vi "AlliGator Compute Interpolated Color Map (Multipoints).vi"(7 "Background Color":u32(colorbox), 8 "Error In":errorcluster, 9 "Decay Range Exponent":dbl=1.0, 10 "Color Array":u32[](array[numeric]), 11 "XY Graph":refnum<vi>) -> (0 "Error Out":errorcluster, 3 "Vertices":cluster{"X":dbl, "Y":dbl}[](array[cluster]))   [LabVIEW 2021, in "AlliGator Phasor Plot Color Map.lvlib"]
doc: "Computes a color map based on user-provided parameters."
uses:
  <vilib>/Utility/error.llb/DialogType.ctl
  <vilib>/picture/picture.llb/imagedata.ctl
  <vilib>/Analysis/geometry.llb/Point in Polygon (Scalar).vi
  AlliGator Phasor Plot Color Map.lvlib
  Image/Image.lvlib
  <vilib>/vision/NI_Vision_Development_Module.lvlib
  <vilib>/Analysis/NI_AAL_Geometry.lvlib
  Time/Time.lvlib
panel:
  out "CPU (s)":dbl
  # "see the AlliGator License on the block diagram (Ctrl+E or Window:Show Block Diagram)"
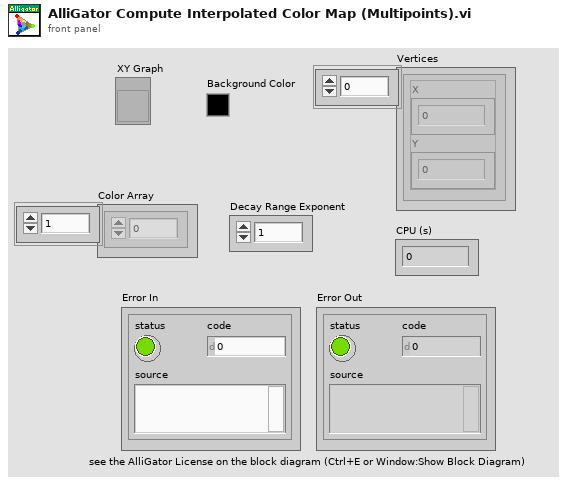
[diagram p1: front panel]
types:
  T1 = typedef "LVCursorListTypeDef.ctl" = cluster{"Name":string, "Color":u32, "Style":u8, "Point Style":u8, "Name Visible":bool, "Allow Drag":bool, "Cursor Mode":u32, "Plot":i32, "Index":i32, "Position":cluster{"X":dbl, "Y":dbl}, "X Scale":u32, "Y Scale":u32, "Watch Plots":i32[], "Watch All Plots":bool, "Plot Area":i32, "Label Offset":cluster{"X":dbl, "Y":dbl}}[]
  T2 = typedef "LVBoundsTypeDef.ctl" = cluster{"Width":u32, "Height":u32}
  T3 = typedef "LVRectTypeDef.ctl" = cluster{"Left":i16, "Top":i16, "Right":i16, "Bottom":i16}
  T4 = cluster{"left":i16, "top":i16, "right":i16, "bottom":i16}
  T5 = typedef "imagedata.ctl" = cluster{"image type":i32, "image depth":i32, "image":u8[], "mask":u8[], "colors":u32[], "Rectangle":cluster{"left":i16, "top":i16, "right":i16, "bottom":i16}}
  T6 = typedef "DialogType.ctl" = u16
  T7 = typedef "LVPoint32TypeDef.ctl" = cluster{"Horizontal":i32, "Vertical":i32}
  T8 = cluster{"Red (or Hue) value":u8, "Green (or Sat) value":u8, "Blue (or Light or Val) value":u8}[]
  T9 = typedef "NI_AAL_Geometry.lvlib/Point in Polygon Position.ctl" = u16
  T10 = cluster{"Red (or Hue) value":u8, "Green (or Sat) value":u8, "Blue (or Light or Val) value":u8}
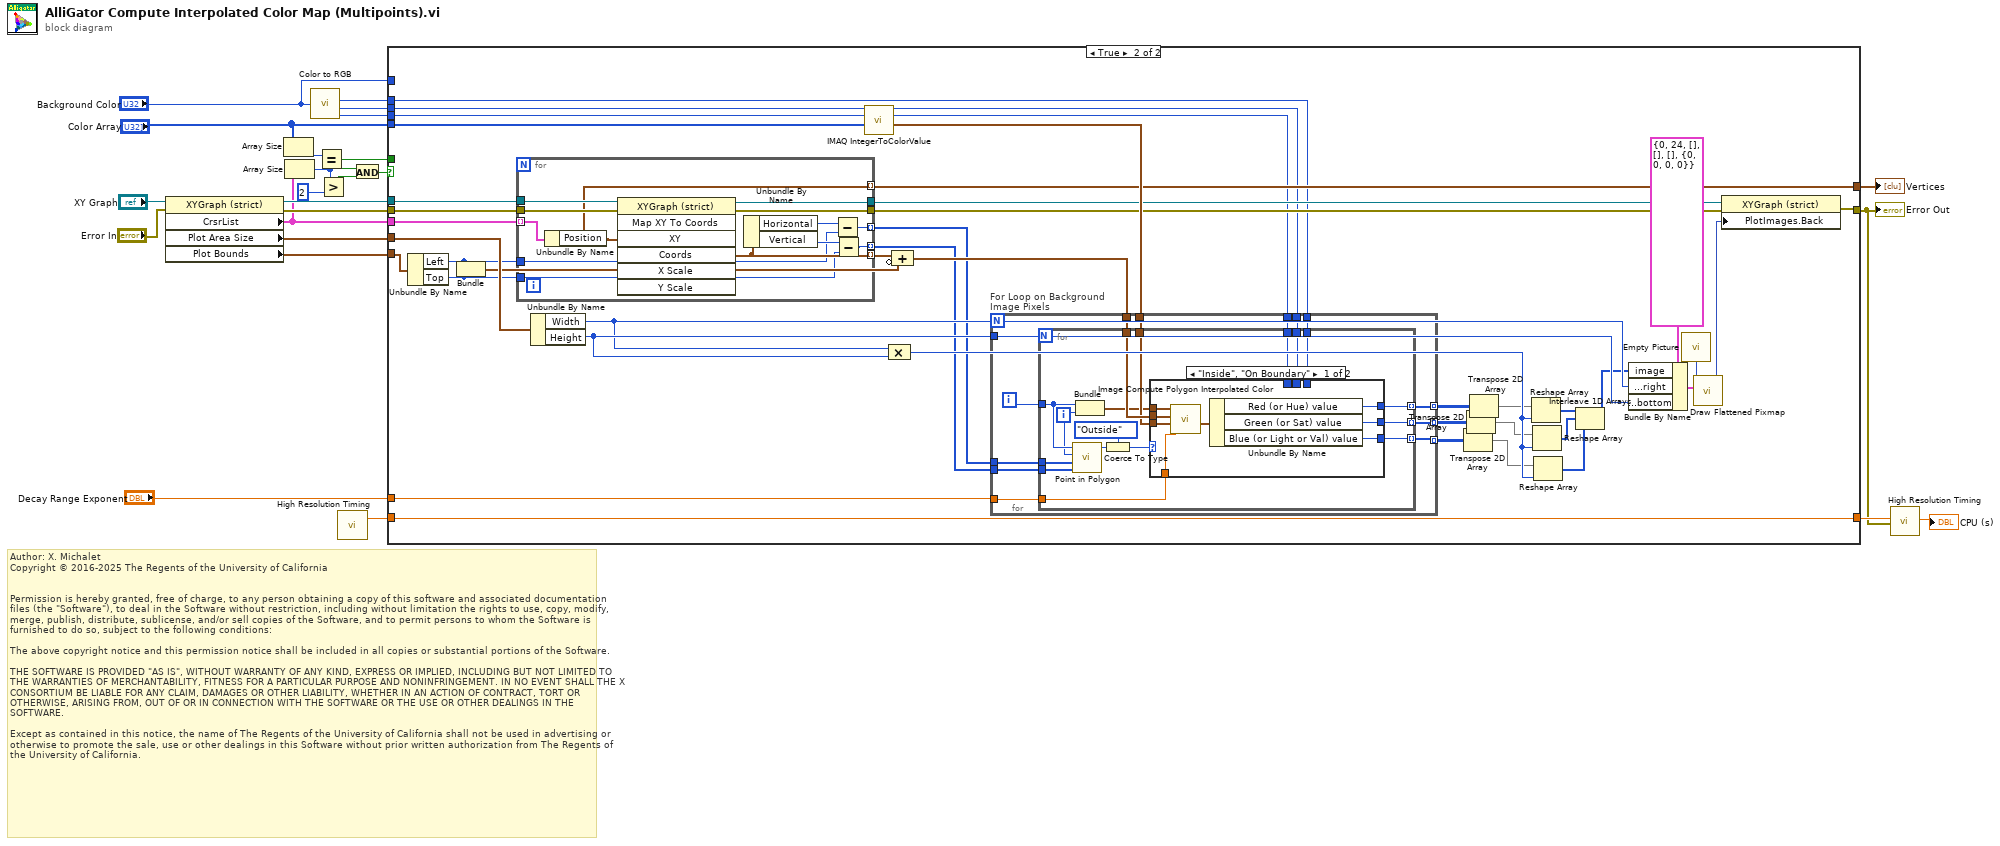
[diagram p0: block diagram]
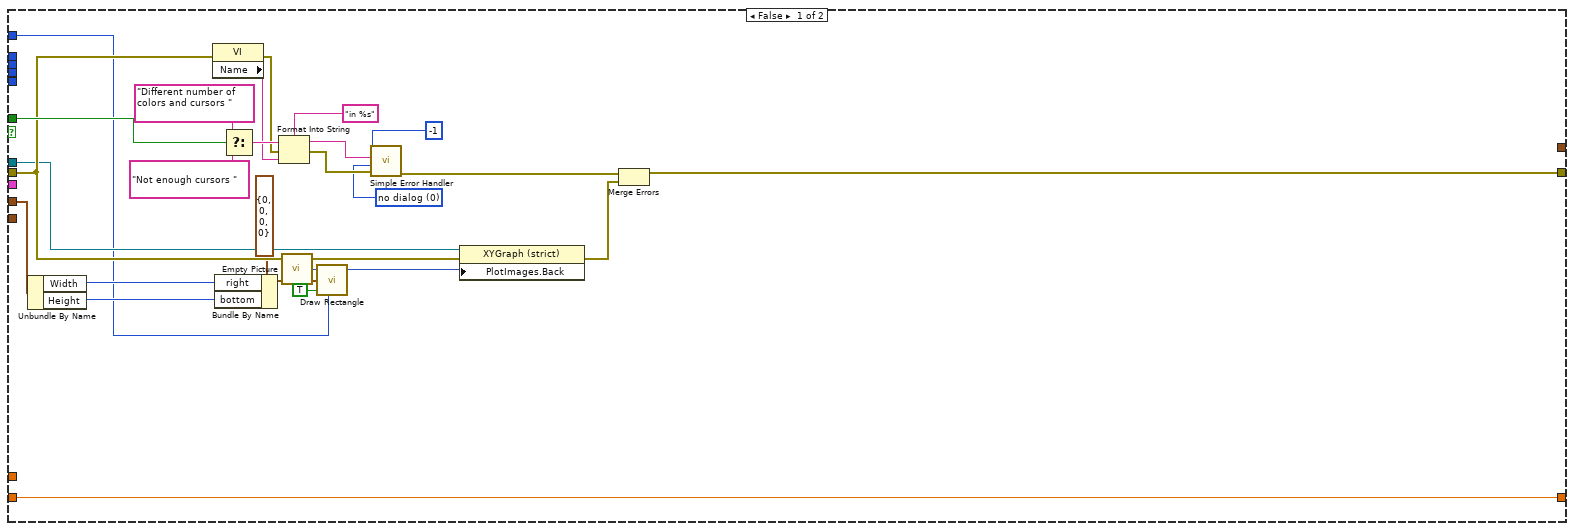
[diagram p2: hidden frame]
diagram:
  # "Author: X. Michalet\nCopyright © 2016-2025 The Regents of the University of California\n \n\nPermission is hereby granted, free of charge, to any person obtaining a copy of this software and associated documentation files (the \"Software\"), to deal in the Software without restriction, including without limitation the rights to use, copy, modify, merge, publish, distribute, sublicense, and/or sell copies of the Software, and to permit persons to whom the Software is furnished to do so, subject to the following conditions:\n\nThe above copyright notice and this permission notice shall be included in all copies or substantial portions of the Software.\n\nTHE SOFTWARE IS PROVIDED \"AS IS\", WITHOUT WARRANTY OF ANY KIND, EXPRESS OR IMPLIED, INCLUDING BUT NOT LIMITED TO THE WARRANTIES OF MERCHANTABILITY, FITNESS FOR A PARTICULAR PURPOSE AND NONINFRINGEMENT. IN NO EVENT SHALL THE X CONSORTIUM BE LIABLE FOR ANY CLAIM, DAMAGES OR OTHER LIABILITY, WHETHER IN AN ACTION OF CONTRACT, TORT OR OTHERWISE, ARISING FROM, OUT OF OR IN CONNECTION WITH THE SOFTWARE OR THE USE OR OTHER DEALINGS IN THE SOFTWARE.\n\nExcept as contained in this notice, the name of The Regents of the University of California shall not be used in advertising or otherwise to promote the sale, use or other dealings in this Software without prior written authorization from The Regents of the University of California."
  n1 = property class="XYGraph (strict)"(reference="XY Graph", error in="Error In") -> (reference out=w22:refnum<vi>, error out=w21:errorcluster, "CrsrList"=w19:T1, "Plot Area Size"=w20:T2, "Plot Bounds"=w11:T3)
  n2 = Array Size(array="Color Array") -> (size(s)=w18:i32)
  n3 = Array Size(array=w19) -> (size(s)=w17:i32)
  n4 = call <vilib>:"Color to RGB.vi"("Color"="Background Color") -> ("R"=w5:u8, "G"=w4:u8, "B"=w3:u8)  [unwired: 1 out]
  n5 = Equal?(x=w18, y=w17) -> (x = y?=w13:bool)
  n6 = Greater?(x=w17, y=2) -> (0:w15:bool)
  n7 = call "High Resolution Timing.vi"() -> ("relative seconds"=w9:dbl)  [unwired: 17 in, 2 out]
  n8 = And(x=w13, y=w15) -> (x .and. y?=w14:bool)
  n9 = case shown="True" w14 {
    tunnel: w22 -> [w37 w90]
    tunnel: w21 -> [w38 w89]
    tunnel: w20 -> [w36 w88]
    tunnel: w19 -> [_ w87]
    tunnel: w13 -> [w50 _]
    tunnel: [w34 w61] -> w6
    tunnel: "Color Array" -> [_ w85]
    tunnel: w11 -> [_ w70]
    tunnel: [_ w56] -> w10
    tunnel: w9 -> [w35 w55]
    tunnel: [w35 w55] -> w8
    tunnel: w5 -> [_ w54]
    tunnel: w4 -> [_ w53]
    tunnel: w3 -> [_ w52]
    tunnel: "Background Color" -> [w26 _]
    tunnel: "Decay Range Exponent" -> [_ w51]
    frame False {
      w40 = T6 0 items=["no dialog", "OK message", "continue or stop message", "OK message + warnings", "continue/stop + warnings"] ("type of dialog (OK msg:1)")
      n10 = Unbundle By Name(w36) -> ("Width"=w28:u32, "Height"=w27:u32)
      n11 = property class="VI"(error in=w38) -> (error out=w43:errorcluster, "Name"=w44:string)  [unwired: 1 in, 1 out]
      n12 = Bundle By Name(cluster=T4 {"left"=0, "top"=0, "right"=0, "bottom"=0} ("rect"), "right"=w28, "bottom"=w27) -> (w29:T4)
      n13 = Select(t="Different number of colors and cursors " ("error source (\" \")"), s=w50, f="Not enough cursors " ("error source (\" \")")) -> (s? t:f=w47:string)
      n14 = Format Into String(format string="in %s", initial string=w47, error in=w43, w44) -> (resulting string=w46:string, error out=w42:errorcluster)
      n15 = call "Empty Picture"() -> ("empty picture"=w31:picture)
      n16 = call <vilib>:"Draw Rectangle.vi"("picture"=w31, "rect"=w29, "fill?(F)"=TRUE, "color(black)"=w26) -> ("new picture"=w32:picture)  [unwired: 5 in]
      n17 = call <vilib>:"Simple Error Handler.vi"("error code (no error:0)"=-1, "error source (\" \")"=w46, "type of dialog (OK msg:1)"=w40, "error in (no error)"=w42) -> ("error out"=w49:errorcluster)  [unwired: 1 in, 4 out]
      n18 = property class="XYGraph (strict)"(reference=w37, error in=w38, "PlotImages.Back"=w32) -> (error out=w33:errorcluster)  [unwired: 1 out]
      n19 = Merge Errors(w49, w33) -> (w34:errorcluster)
    }
    frame True {
      n20 = Unbundle By Name(w70) -> ("Left"=w59:i16, "Top"=w58:i16)
      n21 = Bundle("Left"=w59, "Top"=w58) -> (w57:cluster{"Left":i16, "Top":i16})  [unwired: 1 in]
      n22 = for {
        tunnel: w87 -> [w144] mode=indexing
        tunnel: w90 -> [w143]
        tunnel: w89 -> [w142]
        tunnel: [w140] -> w86 mode=indexing
        tunnel: [w141] -> w62
        tunnel: [w137] -> w69 mode=indexing
        tunnel: [w136] -> w68 mode=indexing
        tunnel: [w135] -> w63
        tunnel: w59 -> [w134]
        tunnel: w58 -> [w133]
        tunnel: [w132] -> w56 mode=indexing
        n23 = Unbundle By Name(w144) -> ("Position"=w132:cluster{"X":dbl, "Y":dbl})
        n24 = invoke class="XYGraph (strict)" method="Map XY To Coords"(reference=w143, error in=w142, "XY"=w132) -> (reference out=w135:refnum<vi>, error out=w141:errorcluster, "Coords"=w140:T7)  [unwired: 4 in, 4 out]
        n25 = Unbundle By Name(w140) -> ("Horizontal"=w139:i32, "Vertical"=w138:i32)
        n26 = Subtract(x=w139, y=w134) -> (x-y=w137:i32)
        n27 = Subtract(x=w138, y=w133) -> (x-y=w136:i32)
      }
      n28 = Unbundle By Name(w88) -> ("Width"=w71:u32, "Height"=w73:u32)
      n29 = call "IMAQ IntegerToColorValue"("1D U32 array"=w85) -> ("1D Color value array"=w84:T8)  [unwired: 4 in, 3 out]
      n30 = Compound Arithmetic op=MULTIPLY(w71, w73) -> (w72:u32)
      n31 = Compound Arithmetic op=ADD(w86, invert w57) -> (w83:T7[])
      n32 = for "For Loop on Background Image Pixels" {
        N: w71 -> [_]
        tunnel: w73 -> [w103]
        tunnel: w83 -> [w102]
        tunnel: w84 -> [w101]
        tunnel: [w99] -> w79 mode=indexing
        tunnel: [w98] -> w78 mode=indexing
        tunnel: [w97] -> w77 mode=indexing
        tunnel: w69 -> [w96]
        tunnel: w68 -> [w95]
        tunnel: w51 -> [w94]
        tunnel: w54 -> [w93]
        tunnel: w53 -> [w92]
        tunnel: w52 -> [w91]
        i -> [w100]
        n33 = for {
          N: w103 -> [_]
          tunnel: w102 -> [w120]
          tunnel: w101 -> [w119]
          tunnel: w100 -> [w113]
          tunnel: [w117] -> w99 mode=indexing
          tunnel: [w116] -> w98 mode=indexing
          tunnel: [w115] -> w97 mode=indexing
          tunnel: w96 -> [w111]
          tunnel: w95 -> [w110]
          tunnel: w94 -> [w109]
          tunnel: w93 -> [w106]
          tunnel: w92 -> [w105]
          tunnel: w91 -> [w104]
          i -> [w112]
          n34 = call-poly <vilib>:"Point in Polygon.vi"("Polygon Y"=w110, "Polygon X"=w111, "y"=w112, "x"=w113) -> ("position"=w114:T9)  [unwired: 6 in, 1 out]
          n35 = Bundle(w113, w112) -> (w118:cluster{i32, i32})  [unwired: 1 in]
          n36 = Coerce To Type(0:w114, 1:enum16{"Inside", "On Boundary", "Outside"}."Outside") -> (2:w107:enum16{"Inside", "On Boundary", "Outside"})
          n37 = case shown="\"Inside\", \"On Boundary\"" w107 {
            tunnel: w120 -> [w128 _]
            tunnel: w119 -> [w127 _]
            tunnel: w118 -> [w126 _]
            tunnel: [w124 w131] -> w117
            tunnel: [w123 w130] -> w116
            tunnel: [w122 w129] -> w115
            tunnel: w109 -> [w121 _]
            tunnel: w106 -> [_ w131]
            tunnel: w105 -> [_ w130]
            tunnel: w104 -> [_ w129]
            frame "Inside", "On Boundary" {
              n38 = call "Image Compute Polygon Interpolated Color.vi"("Decay Range Exponent"=w121, "1D Color value array"=w127, "Vertices"=w128, "Pixel"=w126) -> ("Color Components"=w125:T10)  [unwired: 6 in, 1 out]
              n39 = Unbundle By Name(w125) -> ("Red (or Hue) value"=w124:u8, "Green (or Sat) value"=w123:u8, "Blue (or Light or Val) value"=w122:u8)
            }
            frame "Outside" {
            }
          }
        }
      }
      n40 = Transpose 2D Array(2D array=w77) -> (transposed array=w64:u8[][])
      n41 = Transpose 2D Array(2D array=w78) -> (transposed array=w65:u8[][])
      n42 = Transpose 2D Array(2D array=w79) -> (transposed array=w66:u8[][])
      n43 = Reshape Array(w66, w72) -> (w76:u8[])
      n44 = Reshape Array(w65, w72) -> (w75:u8[])
      n45 = Reshape Array(w64, w72) -> (w74:u8[])
      n46 = Interleave 1D Arrays(w76, w75, w74) -> (w67:u8[])
      n47 = Bundle By Name(cluster=T5 {"image type"=0, "image depth"=24, "image"=[], "mask"=[], "colors"=[], "Rectangle"={"left"=0, "top"=0, "right"=0, "bottom"=0}} ("image data"), "image"=w67, "Rectangle.right"=w71, "Rectangle.bottom"=w73) -> (w80:T5)
      n48 = call "Empty Picture"() -> ("empty picture"=w82:picture)
      n49 = call <vilib>:"Draw Flattened Pixmap.vi"("image data"=w80, "picture"=w82) -> ("new picture"=w60:picture)  [unwired: 7 in]
      n50 = property class="XYGraph (strict)"(reference=w63, error in=w62, "PlotImages.Back"=w60) -> (error out=w61:errorcluster)  [unwired: 1 out]
    }
  }
  "Error Out" <- w6
  "Vertices" <- w10
  n51 = call "High Resolution Timing.vi"("relative seconds (NaN)"=w8, "Error In"=w6) -> ("elapsed (relative) seconds"=→"CPU (s)":dbl)  [unwired: 15 in, 2 out]
